vi "FTW-CodeGen-OnResize2.vi"(0 "State In":T3, 5 "XRef":refnum<vi>, 7 "Bounds":T2, 9 "Mouse Mods":T1) -> (4 "State Out":T3, 6 "Reply":string[](array[string]))   [LabVIEW 2015, in "FTW-Dataflow-Synchronizer.xnode"]
uses:
  FTW-Dataflow-Synchronizer.xnode
  FTW-CodeGen-State.ctl
  FTW-CodeGen-XNodeReplyType.ctl
panel:
  # "Inputs"
  # "Outputs"
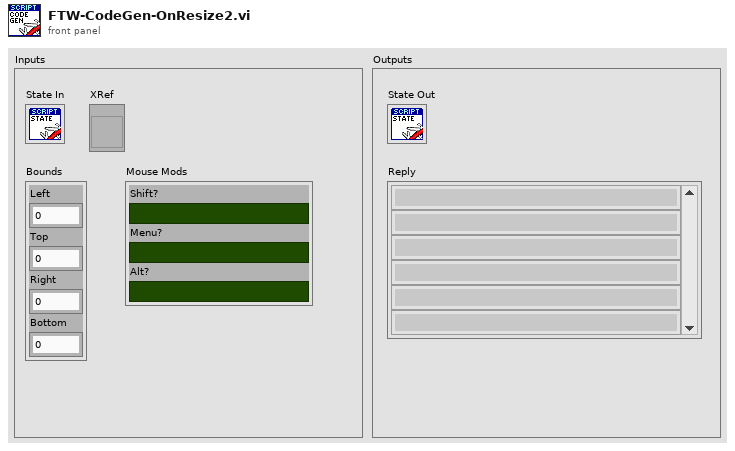
[diagram p1: front panel]
types:
  T1 = cluster{"Shift?":bool, "Menu?":bool, "Alt?":bool}
  T2 = cluster{"Left":i32, "Top":i32, "Right":i32, "Bottom":i32}
  T3 = typedef "FTW-Dataflow-Synchronizer.xnode/FTW-CodeGen-State.ctl" = cluster{"InputTerminals":cluster{"Wired?":bool, "ID":string, "DataName":string, "DataColor":u32, "Type":variant}[], "EnableTiming?":bool}
  T4 = typedef "FTW-CodeGen-XNodeReplyType.ctl" = enum16{"NoReply", "ForceAdaptToInputs", "UpdateTerms", "GenCode", "GenCode+CosmeticUpdate"}
  T5 = cluster{"Wired?":bool, "ID":string, "DataName":string, "DataColor":u32, "Type":variant}[]
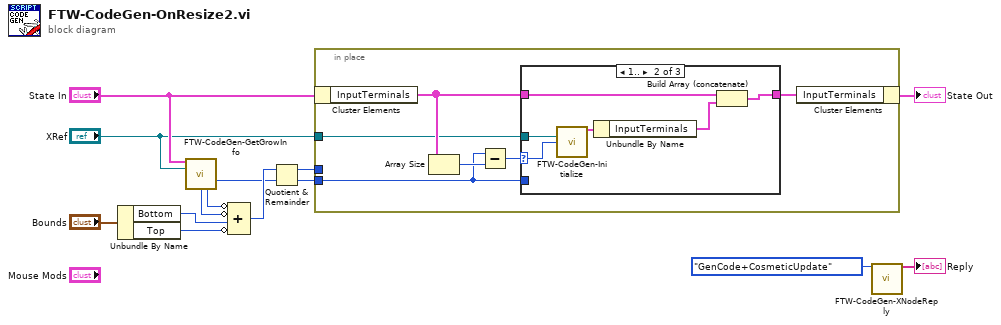
[diagram p0: block diagram]
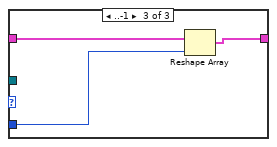
[diagram p3: hidden frame]
diagram:
  n1 = Unbundle By Name("Bounds") -> ("Bottom"=w13:i32, "Top"=w12:i32)
  n2 = call "FTW-CodeGen-GetGrowInfo.vi"("State In"="State In", "XRef"="XRef") -> ("Terminal Height"=w8:i32, "Bottom Banner Height"=w10:i32, "Total Top Banner Height"=w11:i32)  [unwired: 5 in, 6 out]
  n3 = Compound Arithmetic op=ADD(invert w11, invert w10, w13, invert w12) -> (w9:i32)
  n4 = Quotient & Remainder(x=w9, y=w8) -> (x-y*floor(x/y)=w3:i32, floor(x/y)=w5:i32)
  n5 = in-place {
    in-place-border: w5 -> [w17]
    in-place-border: "XRef" -> [w15]
    in-place-border: w3 -> [_]
    n6 = in-place-cluster #1("State In") -> ("InputTerminals"=w19:T5)
    n7 = Array Size(array=w19) -> (size(s)=w18:i32)
    n8 = Subtract(x=w17, y=w18) -> (x-y=w16:i32)
    n9 = case shown="1.." w16 {
      selector: w16 -> [_ w26 _]
      tunnel: [w21 w24 w30] -> w20
      tunnel: w19 -> [w21 w27 w29]
      tunnel: w17 -> [_ _ w28]
      tunnel: w15 -> [_ w25 _]
      frame 0 {
      }
      frame 1.. {
        n10 = call "FTW-CodeGen-Initialize.vi"("XRef"=w25, "Items"=w26) -> ("State Out"=w23:T3)  [unwired: 13 in]
        n11 = Unbundle By Name(w23) -> ("InputTerminals"=w22:T5)
        n12 = Build Array (concatenate)(w27, w22) -> (w24:T5)
      }
      frame ..-1 {
        n13 = Reshape Array(w29, w28) -> (w30:T5)
      }
    }
    n14 = in-place-cluster #1("InputTerminals"=w20) -> (→"State Out":T3)
  }
  n15 = call "FTW-CodeGen-XNodeReply.vi"("XNode Reply Type"=FTW-CodeGen-XNodeReplyType."GenCode+CosmeticUpdate") -> ("Reply"=→"Reply":string[])  [unwired: 14 in]
